vi "StartMeasurement.vi"(0 "a_hDevice":i32, 5 "a_hWnd":i32, 7 "a_Nmsr":i16, 11 "MeasConfigType":T1) -> (8 "Status":string, 15 "StartTime":u32)   [LabVIEW 2016]
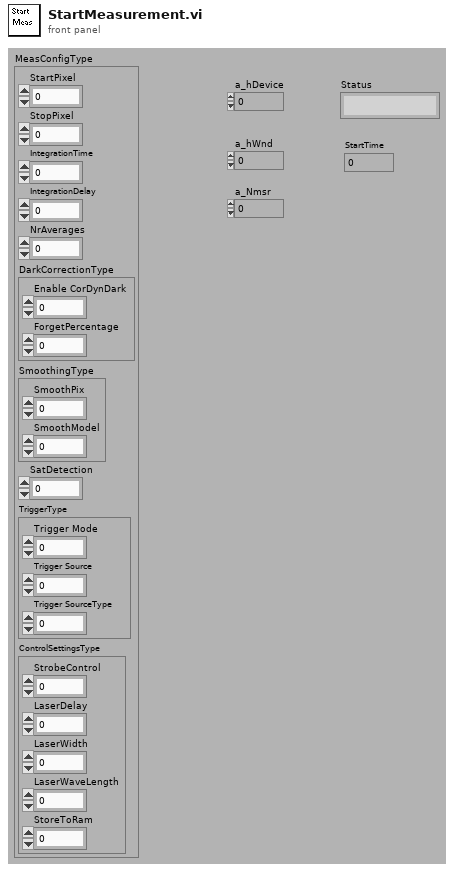
[diagram p1: front panel]
types:
  T1 = cluster{"StartPixel":u16, "StopPixel":u16, "IntegrationTime":sgl, "IntegrationDelay":u32, "NrAverages":u32, "DarkCorrectionType":cluster{"Enable CorDynDark":u8, "ForgetPercentage":u8}, "SmoothingType":cluster{"SmoothPix":u16, "SmoothModel":u8}, "SatDetection":u8, "TriggerType":cluster{"Trigger Mode":u8, "Trigger Source":u8, "Trigger SourceType":u8}, "ControlSettingsType":cluster{"StrobeControl":u16, "LaserDelay":u32, "LaserWidth":u32, "LaserWaveLength":sgl, "StoreToRam":u16}}
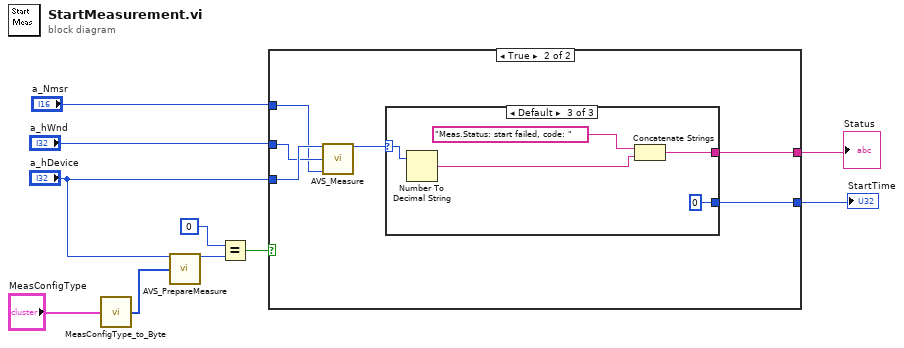
[diagram p0: block diagram]
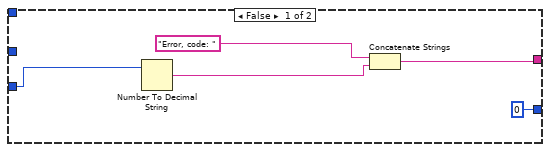
[diagram p2: hidden frame]
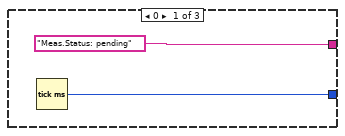
[diagram p3: hidden frame]
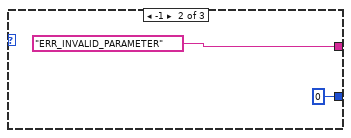
[diagram p4: hidden frame]
diagram:
  n1 = call "MeasConfigType_to_Byte.vi"("MeasConfigType"="MeasConfigType") -> ("Byte Array"=w1:u8[])  [unwired: 4 in]
  n2 = call "AVS_PrepareMeasure.vi"("a_hDevice"="a_hDevice", "MeasConfArray"=w1) -> ("Output Value"=w9:i32)  [unwired: 13 in]
  n3 = Equal?(x=u8 0, y=w9) -> (x = y?=w8:bool)
  n4 = case shown="True" w8 {
    tunnel: "a_hDevice" -> [w13 w21]
    tunnel: "a_hWnd" -> [_ w20]
    tunnel: "a_Nmsr" -> [_ w19]
    tunnel: [w12 w17] -> w4
    tunnel: [u32 0 ("millisecond timer value") w16] -> w3
    frame False {
      n5 = Number To Decimal String(number=w13) -> (decimal integer string=w15:string)  [unwired: 1 in]
      n6 = Concatenate Strings("Error, code: ", w15) -> (w12:string)
    }
    frame True {
      n7 = call "AVS_Measure.vi"("a_hDevice"=w21, "a_hWnd"=w20, "a_Nmsr"=w19) -> ("Output Value"=w18:i32)  [unwired: 12 in]
      n8 = case shown="Default" w18 {
        selector: w18 -> [_ _ w30]
        tunnel: ["Meas.Status: pending" "ERR_INVALID_PARAMETER" w27] -> w17
        tunnel: [w22 u32 0 ("millisecond timer value") u32 0 ("millisecond timer value")] -> w16
        frame 0 {
          n9 = Tick Count (ms)() -> (millisecond timer value=w22:u32)
        }
        frame -1 {
        }
        frame Default {
          n10 = Number To Decimal String(number=w30) -> (decimal integer string=w29:string)  [unwired: 1 in]
          n11 = Concatenate Strings("Meas.Status: start failed, code: ", w29) -> (w27:string)
        }
      }
    }
  }
  "Status" <- w4
  "StartTime" <- w3
